vi "JGPR4_Bug_PID.vi"() -> ()   [LabVIEW 2019]
doc: "This is the Main VI for the bug PID controller.\n\nIt allows the user to modify and verify the temperature control parameters at the beginning, and then starts temperature control to obtain the desired setpoint. The user can choose manual power control at any time during operation as well. It also allows the user to create a temperature log file that logs the temperature control details for each cycle during the experiment. This can be quite useful to analyze and refine the control parameters later on, or help understand why experiments might get off track in the middle of the night.\n\nJuan Gamez\nP3600\nCSUSB Physics"
uses:
  components/typedefs/exp sequence.ctl
  components/typedefs/scale control.ctl
  components/typedefs/temp indicator.ctl
  components/typedefs/temp control status.ctl
  components/typedefs/PID control parameters.ctl
  components/typedefs/PID exec cluster.ctl
  components/typedefs/bug temp file info.ctl
  components/typedefs/temp mode enum.ctl
  components/globals/Bug temp globals.vi
panel:
  out "exit loc":bool
  in  "Monitor":T1(tab)
  in  "Scale Control":T2
  out "T cont status":T3={"Control status"=enum."In Control Band", "Temp"=31.819617943507183, "Power"=0.0622151359889699, "Time in settle band"=0.0, "Settled"=FALSE, "Low"=FALSE, "High"=FALSE, "Setpoint"=30.0, "Control"=TRUE, "In Settle Band"=FALSE} caption="Temperature Control Status" {"Setpoint" format="%_6g"; "Power" format="%_6g"; "Temp" format="%_6g"}
  out "Temperature Chart":T5(graph)={"temp out"=31.819617943507183, 30.0, 32.0, 28.0, 30.5, 29.5, 7.465816318676388}
  out "Manual Temp control":bool=TRUE
  out "Setpoint (C)":dbl=30.0
  out "meas index":i32
  in  "clear chart":bool
  out "logging temp":bool
  out "temp log file path":path
  out "Temperature Graph":cluster{"t hist":dbl[], "T hist":dbl[]}[](graph)=[{"t hist"=[0.681, 1.01, 1.338, 1.667, 1.996, 2.323, 2.651, 2.979, 3.308, 3.636, 3.966, 4.294, 4.622, 4.95, 5.282, 5.614, 5.949, 6.292, 6.624, 6.956, 7.29, 7.629, 7.962, 8.298, 8.632, 8.961, 9.305, 9.649, 9.982, 10.321], "T hist"=[28.221637848568264, 28.335463471473247, 28.45177291236797, 28.578054212374127, 28.712611988419383, 28.84616557500516, 28.98818760788282, 29.12927903863408, 29.273265947327218, 29.420201611602806, 29.566232905582694, 29.70936480151545, 29.857453821818012, 29.996629768200933, 30.14076143529155, 30.28185384495856, 30.41983725429435, 30.556691662116748, 30.68413877422978, 30.810295121327613, 30.930958632049965, 31.052323535552546, 31.161736118199713, 31.269603761681765, 31.37376795546072, 31.474170088455764, 31.568601926879808, 31.65482002616045, 31.741394285589706, 31.819617943507183]}, {"t hist"=[0.681, 1.01, 1.338, 1.667, 1.996, 2.323, 2.651, 2.979, 3.308, 3.636, 3.966, 4.294, 4.622, 4.95, 5.282, 5.614, 5.949, 6.292, 6.624, 6.956, 7.29, 7.629, 7.962, 8.298, 8.632, 8.961, 9.305, 9.649, 9.982, 10.321], "T hist"=[61.64927318018057, 60.87935633362467, 59.91081367089514, 59.07163506893572, 58.05431280608125, 56.97210065484677, 55.985935993807566, 54.81990049342825, 53.76683173570311, 52.62763554543207, 51.438400944419776, 50.316274027152325, 49.20160602426924, 47.947916986672055, 46.929584951781365, 45.70234026722682, 44.56571400351665, 43.46069894631547, 42.34612964276051, 41.30873367322221, 40.22693480489379, 39.23489588337625, 38.167150974118684, 37.28797871837572, 36.32680632996466, 35.39340435832317, 34.47125846281813, 33.68091084957889, 32.922923294982894, 32.02199191964152]}]
  out "Exp Seq":T6 caption="Experimental Sequence"
  in  "create T log":bool
  out "temp log file path":path
  in  "Default Set":dbl=30.0 caption="Default Setpoint (C)"
  in  "Set T cont params":bool
  out "T Cont Params":T7={"Setpoint"=30.0, "Control Bandwidth"=4.0, "Integral Time"=30.0, "Int\nON"=TRUE, "Derivative Tme"=0.5, "Der\nON"=TRUE, "Settle Bandwidth"=1.0, "Settle Time"=60.0} caption="Temp Control Parameters" {"Settle Time" step=1.0; "Settle Bandwidth" step=0.01; "Derivative Tme" step=0.01; "Integral Time" step=1.0; "Control Bandwidth" step=0.1; "Setpoint" step=0.1}
  out "T log file exists":bool
  in  "proceed":bool
  in  "exit":bool
  in  "exit":bool
  in  "Setpoint (C)":dbl=30.0
  out "Data being logged":bool
  out "Total elapsed time (s)":i32=10
  out "T Cont Params":T7={"Setpoint"=30.0, "Control Bandwidth"=4.0, "Integral Time"=30.0, "Int\nON"=TRUE, "Derivative Tme"=0.5, "Der\nON"=TRUE, "Settle Bandwidth"=1.0, "Settle Time"=60.0} caption="Temp Control Parameters" {"Settle Time" step=1.0; "Settle Bandwidth" step=0.01; "Derivative Tme" step=0.01; "Integral Time" step=1.0; "Control Bandwidth" step=0.1; "Setpoint" step=0.1}
  in  "Mod T cont":bool
  in  "Manual Power":dbl(slide) scale=0.0..1.0
  in  "Manual Control":bool
  # "Bug Experiment \nPID Temperature Control"
  # "Note: This TAB is under system control, the others are under user control"
  # "Experiment Completed"
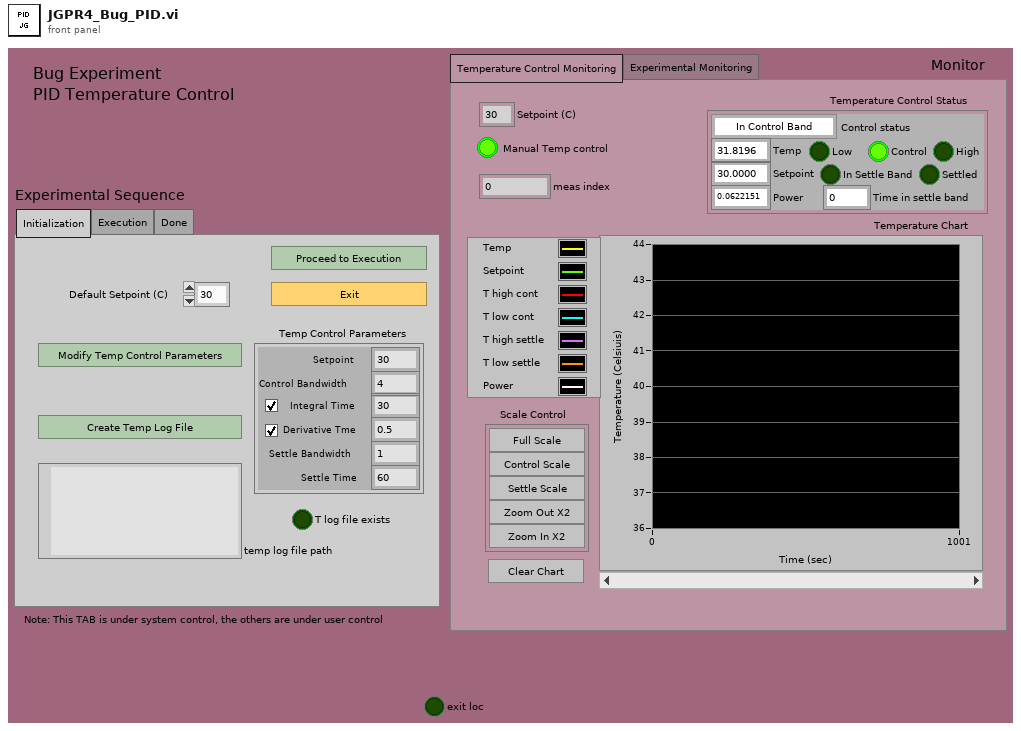
[diagram p1: front panel]
types:
  T1 = enum32{"Temperature Control Monitoring", "Experimental Monitoring"}
  T2 = typedef "scale control.ctl" = cluster{"Full Scale":bool, "Control Scale":bool, "Settle Scale":bool, "Zoom Out X2":bool, "Zoom In X2":bool}
  T3 = typedef "temp indicator.ctl" = cluster{"Control status":T4, "Temp":dbl, "Power":dbl, "Time in settle band":dbl, "Settled":bool, "Low":bool, "High":bool, "Setpoint":dbl, "Control":bool, "In Settle Band":bool}
  T4 = typedef "temp control status.ctl" = enum16{"In Settle Band", "In Control Band", "Below Control Band", "Above Control Band"}
  T5 = cluster{"temp out":dbl, dbl, dbl, dbl, dbl, dbl, dbl}
  T6 = typedef "exp sequence.ctl" = enum32{"Initialization", "Execution", "Done"}
  T7 = typedef "PID control parameters.ctl" = cluster{"Setpoint":dbl, "Control Bandwidth":dbl, "Integral Time":dbl, "Int\nON":bool, "Derivative Tme":dbl, "Der\nON":bool, "Settle Bandwidth":dbl, "Settle Time":dbl}
  T8 = cluster{"temp out":dbl, dbl, dbl, dbl, dbl, dbl, dbl}[]
  T9 = typedef "temp mode enum.ctl" = enum16{"Setting up", "Listening to exec", "Exit"}
  T10 = typedef "PID exec cluster.ctl" = cluster{"T log file":T11, "error":errorcluster, "elapsed time (s)":dbl}
  T11 = typedef "bug temp file info.ctl" = cluster{"log exists":bool, "File refnum":refnum<file>, "temp log file path":path}
  T12 = typedef "temp cont cluster.ctl" = cluster{"exec":T13, "T status":T3, "T params":T7, "utility":T14}
  T13 = typedef "temp exec cluster.ctl" = cluster{"T mode":T9, "exec setpoint":dbl, "reset":bool, "man power":dbl, "man":bool, "log":bool, "clear":bool}
  T14 = typedef "temp cont utility.ctl" = cluster{"meas index":i32, "wait (ms)":i32, "H Vmax":dbl, "power out":dbl, "heat volt out":dbl, "heat volt in":dbl, "therm volt":dbl, "t T P hist":dbl[][], "cont hist":dbl[][]}
  T15 = typedef "DAQ T state cluster.ctl" = cluster{"DAQ state":T16, "device":tag, "start (ms)":i32, "error":errorcluster, "T cont":T12}
  T16 = typedef "DAQ T state enum.ctl" = enum16{"Global comm", "Meas T & P", "PID power calc", "Man Power set", "Output Power", "Wait", "Exit"}
  T17 = cluster{"Temp":dbl, "Setpoint":dbl, "THC":dbl, "TLC":dbl, "THS":dbl, "TLS":dbl, dbl}
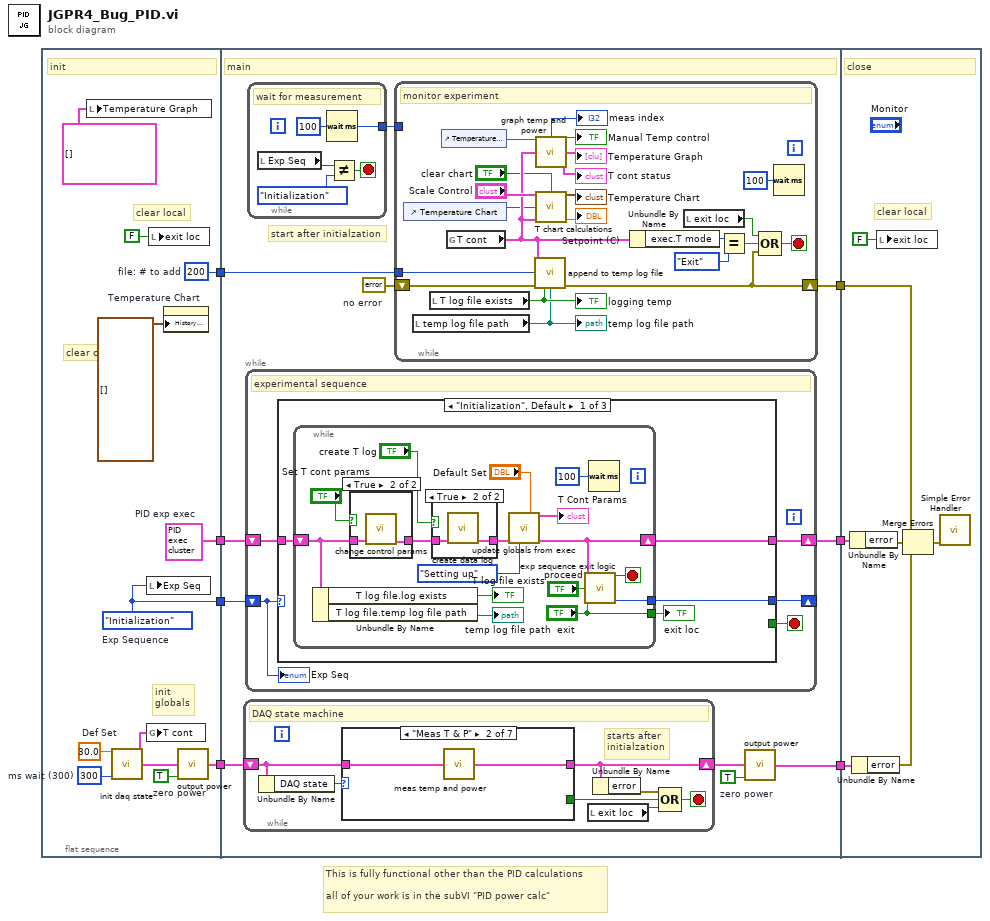
[diagram p0: block diagram]
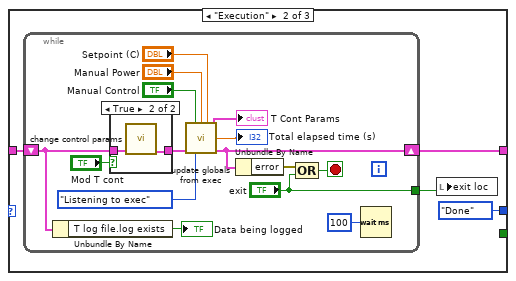
[diagram p4: hidden frame]
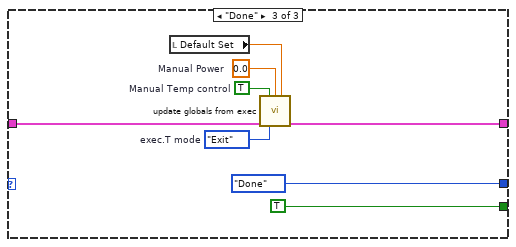
[diagram p6: hidden frame]
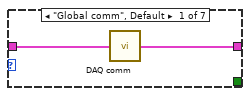
[diagram p7: hidden frame]
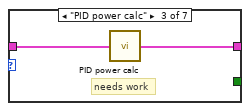
[diagram p8: hidden frame]
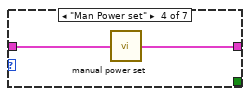
[diagram p9: hidden frame]
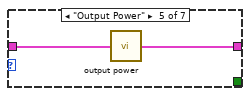
[diagram p10: hidden frame]
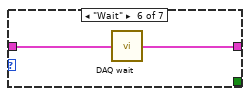
[diagram p11: hidden frame]
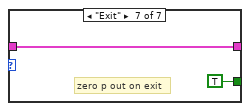
[diagram p12: hidden frame]
diagram:
  # "This is fully functional other than the PID calculations\n\nall of your work is in the subVI \"PID power calc\""
  n1 = flat-sequence {
    tunnel: [w10] -> w4
    tunnel: [w17] -> w3
    tunnel: [w14] -> w2
    tunnel: [w8] -> w1
    tunnel: [w30] -> w7
    tunnel: [w29] -> w6
    tunnel: [w22] -> w5
    tunnel: w4 -> [w28]
    tunnel: w3 -> [w27]
    tunnel: w2 -> [w26]
    tunnel: w1 -> [w20]
    tunnel: w7 -> [w143]
    tunnel: w6 -> [w142]
    tunnel: w5 -> [w141]
    frame #0 {
      w8 = 200  # file: # to add
      w9 = TRUE  # zero power
      w13 = 30.0  # Def Set
      w17 = T10 {"T log file"={"log exists"=FALSE, "File refnum"=refnum, "temp log file path"=path ""}, "error"={"status"=FALSE, "code"=0, "source"=""}, "elapsed time (s)"=0.0}  # PID exp exec
      w14 = exp_sequence."Initialization"  # Exp Sequence
      w18 = 300  # ms wait (300)
      # "clear chart"
      # "clear local"
      # "init\nglobals"
      # "init"
      n2 = local write "Temperature Graph"(cluster{"t hist":dbl[], "T hist":dbl[]}[] [] ("Temperature Graph")) -> ()
      n3 = call "init daq state.vi"("Default Setpoint (C)"=w13, "T cont wait time (ms)"=w18) -> ("T cont out for global update"=w12:T12, "DAQ state start out"=w11:T15)  [unwired: 12 in]
      n4 = local write "Exp Seq"(w14) -> ()
      n5 = global write "Bug temp globals.vi" "T cont"(w12) -> ()
      n6 = local write "exit loc"(FALSE ("exit")) -> ()
      n7 = property on="Temperature Chart" class="WFChart (strict)"("History Data"=T8 []) -> ()  [unwired: 2 in, 2 out]
      n8 = call "output power.vi"("DAQ state cluster in"=w11, "zero power"=w9) -> ("DAQ state cluster out"=w10:T15)  [unwired: 13 in]
    }
    frame #1 {
      w21 = errorcluster {"status"=FALSE, "code"=0, "source"=""}  # no error
      w24 = TRUE  # zero power
      # "start after initialzation"
      # "main"
      n9 = while {
        shift-right: [w120] -> w23
        shift-left: w28 -> [w121]
        stop <- w124 stop-if-true
        # "starts after \ninitialzation"
        # "DAQ state machine"
        n10 = Unbundle By Name(w121) -> ("DAQ state"=w122:T16)
        n11 = case shown="\"Meas T & P\"" w122 {
          tunnel: [_ _ _ _ _ _ TRUE] -> w123
          tunnel: w121 -> [w127 w129 w131 w133 w135 w137 w138]
          tunnel: [w126 w128 w130 w132 w134 w136 w138] -> w120
          frame "Global comm", Default {
            n12 = call "DAQ comm.vi"("DAQ T state cluster in"=w127) -> ("DAQ T state cluster out"=w126:T15)  [unwired: 14 in]
          }
          frame "Meas T & P" {
            n13 = call "meas temp and power.vi"("DAQ state cluster in"=w129) -> ("DAQ state cluster out"=w128:T15)  [unwired: 14 in]
          }
          frame "PID power calc" {
            # "needs work"
            n14 = call "PID power calc.vi"("DAQ state cluster in"=w131) -> ("DAQ state cluster out"=w130:T15)  [unwired: 14 in]
          }
          frame "Man Power set" {
            n15 = call "manual power set.vi"("DAQ state cluster in"=w133) -> ("DAQ state cluster out"=w132:T15)  [unwired: 14 in]
          }
          frame "Output Power" {
            n16 = call "output power.vi"("DAQ state cluster in"=w135) -> ("DAQ state cluster out"=w134:T15)  [unwired: 14 in]
          }
          frame "Wait" {
            n17 = call "DAQ wait.vi"("DAQ state cluster in"=w137) -> ("DAQ state cluster out"=w136:T15)  [unwired: 14 in]
          }
          frame "Exit" {
            # "zero p out on exit"
          }
        }
        n18 = local read "exit loc"() -> (w119:bool)
        n19 = Unbundle By Name(w120) -> ("error"=w125:errorcluster)
        n20 = Compound Arithmetic op=OR(w125, w123, w119) -> (w124:bool)
      }
      n21 = while {
        shift-right: [w59] -> _
        shift-left: w26 -> [w60]
        shift-right: [w61] -> w30
        shift-left: w27 -> [w62]
        stop <- w58 stop-if-true
        # "experimental sequence"
        n22 = case shown="\"Initialization\", Default" w60 {
          tunnel: w62 -> [w65 w92 w116]
          tunnel: [w66 w91 w115] -> w61
          tunnel: [w64 exp_sequence."Done" ("Experimental Sequence") exp_sequence."Done" ("Experimental Sequence")] -> w59
          tunnel: [_ _ TRUE] -> w58
          frame "Initialization", Default {
            n23 = while {
              shift-right: [w68] -> w66
              shift-left: w65 -> [w74]
              tunnel: [w70] -> w64
              tunnel: ["exit"] -> w63
              stop <- w71 stop-if-true
              n24 = Unbundle By Name(w74) -> ("T log file.log exists"=→"T log file exists":bool, "T log file.temp log file path"=→"temp log file path":path)
              n25 = case shown="True" "Set T cont params" {
                tunnel: w74 -> [w83 w85]
                tunnel: [w83 w84] -> w78
                frame False {
                }
                frame True {
                  n26 = call "change control params.vi"("PID exp exec in"=w85) -> ("PID exp exec in"=w84:T10)  [unwired: 14 in]
                }
              }
              n27 = case shown="True" "create T log" {
                tunnel: w78 -> [w86 w88]
                tunnel: [w86 w87] -> w77
                frame False {
                }
                frame True {
                  n28 = call "create data log.vi"("PID exp exec in"=w88) -> ("PID exp exec out"=w87:T10)  [unwired: 13 in, 1 out]
                }
              }
              n29 = call "update globals from exec.vi"("Setpoint (C)"="Default Set", "PID exp exec"=w77, "exec.T mode"=temp_mode_enum."Setting up") -> ("T params"=→"T Cont Params":T7, "PID exp exec out"=w68:T10)  [unwired: 10 in, 1 out]
              n30 = call "exp sequence exit logic.vi"("PID exp exec in"=w68, "proceed"="proceed", "exit"="exit") -> ("stop loop"=w71:bool, "Experimental Sequence"=w70:T6)  [unwired: 11 in]
              n31 = Wait (ms)(milliseconds to wait=u32 100) -> ()  [unwired: 1 out]
            }
            "exit loc" <- w63
          }
          frame "Execution" {
            n32 = while {
              shift-right: [w98] -> w91
              shift-left: w92 -> [w102]
              tunnel: ["exit"] -> w90
              stop <- w99 stop-if-true
              n33 = Unbundle By Name(w102) -> ("T log file.log exists"=→"Data being logged":bool)
              n34 = case shown="True" "Mod T cont" {
                tunnel: w102 -> [w108 w110]
                tunnel: [w108 w109] -> w107
                frame False {
                }
                frame True {
                  n35 = call "change control params.vi"("PID exp exec in"=w110) -> ("PID exp exec in"=w109:T10)  [unwired: 14 in]
                }
              }
              n36 = call "update globals from exec.vi"("Manual Temp control"="Manual Control", "Manual Power"="Manual Power", "Setpoint (C)"="Setpoint (C)", "PID exp exec"=w107, "exec.T mode"=temp_mode_enum."Listening to exec") -> ("T params"=→"T Cont Params":T7, "Total elapsed time (s)"=→"Total elapsed time (s)":dbl, "PID exp exec out"=w98:T10)  [unwired: 8 in]
              n37 = Unbundle By Name(w98) -> ("error"=w100:errorcluster)
              n38 = Compound Arithmetic op=OR(w100, "exit") -> (w99:bool)
              n39 = Wait (ms)(milliseconds to wait=u32 100) -> ()  [unwired: 1 out]
            }
            n40 = local write "exit loc"(w90) -> ()
          }
          frame "Done" {
            w112 = TRUE  # Manual Temp control
            w113 = 0.0  # Manual Power
            w111 = temp_mode_enum."Exit"  # exec.T mode
            n41 = local read "Default Set"() -> (w114:dbl)
            n42 = call "update globals from exec.vi"("Manual Temp control"=w112, "Manual Power"=w113, "Setpoint (C)"=w114, "PID exp exec"=w116, "exec.T mode"=w111) -> ("PID exp exec out"=w115:T10)  [unwired: 8 in, 2 out]
          }
        }
        "Exp Seq" <- w60
      }
      n43 = while {
        tunnel: [w31] -> w25
        stop <- w32 stop-if-true
        # "wait for measurement"
        n44 = local read "Exp Seq"() -> (w34:T6)
        n45 = Wait (ms)(milliseconds to wait=u32 100) -> (millisecond timer value=w31:u32)
        n46 = Not Equal?(x=w34, y=exp_sequence."Initialization" ("Experimental Sequence")) -> (x != y?=w32:bool)
      }
      n47 = while {
        shift-right: [w50] -> w29
        shift-left: w21 -> [w51]
        tunnel: w25 -> [_]
        tunnel: w20 -> [w36]
        stop <- w53 stop-if-true
        # "monitor experiment"
        n48 = control-ref of="Temperature Chart"() -> (w38:refnum<vi>)
        n49 = local read "temp log file path"() -> (w48:path)
        "temp log file path" <- w48
        n50 = local read "T log file exists"() -> (w49:bool)
        "logging temp" <- w49
        n51 = control-ref of="Temperature Graph"() -> (w39:refnum<vi>)
        n52 = global read "Bug temp globals.vi" "T cont"() -> (w46:T12)
        n53 = call "append to temp log file.vi"("T cont"=w46, "# to add"=w36, "error in (no error)"=w51, "T log file exists"=w49, "temp log file path"=w48) -> ("error out"=w50:errorcluster)  [unwired: 10 in]
        n54 = call "graph temp and power.vi"("Temperature Graph"=w39, "T cont"=w46) -> ("meas index"=→"meas index":i32, "man"=→"Manual Temp control":bool, "T and P graph"=→"Temperature Graph":cluster{"t hist":dbl[], "T hist":dbl[]}[], "T status"=→"T cont status":T3)  [unwired: 10 in]
        n55 = call "T chart calculations.vi"("Scale Control"="Scale Control", "clear chart"="clear chart", "WaveformChart in"=w38, "T cont"=w46) -> ("T chart cluster"=→"Temperature Chart":T17, "Setpoint"=→"Setpoint (C)":dbl)  [unwired: 10 in]
        n56 = Unbundle By Name(w46) -> ("exec.T mode"=w52:T9)
        n57 = local read "exit loc"() -> (w44:bool)
        n58 = Equal?(x=w52, y=temp_mode_enum."Exit" ("exec.T mode")) -> (x = y?=w54:bool)
        n59 = Compound Arithmetic op=OR(w44, w54, w50) -> (w53:bool)
        n60 = Wait (ms)(milliseconds to wait=u32 100) -> ()  [unwired: 1 out]
      }
      n61 = call "output power.vi"("DAQ state cluster in"=w23, "zero power"=w24) -> ("DAQ state cluster out"=w22:T15)  [unwired: 13 in]
    }
    frame #2 {
      # "clear local"
      # "close"
      n62 = Unbundle By Name(w143) -> ("error"=w146:errorcluster)
      n63 = Unbundle By Name(w141) -> ("error"=w145:errorcluster)
      n64 = local write "exit loc"(FALSE ("exit")) -> ()
      n65 = Merge Errors(w142, w146, w145) -> (w144:errorcluster)
      n66 = call <vilib>:"Simple Error Handler.vi"("error in (no error)"=w144) -> ()  [unwired: 4 in, 5 out]
    }
  }
